vi "Write LINX I2C.vi"(8 "error in (no error)":errorcluster, 10 "LINX I2C":refnum<class "LINX I2C.lvclass">, 11 "BMP208 in":refnum<class "BMP208.lvclass">) -> (0 "error out":errorcluster, 3 "BMP208 out":refnum<class "BMP208.lvclass">)   [LabVIEW 2020, in "BMP208.lvclass"]
uses:
  BMP208.lvclass
  LINX I2C/LINX I2C.lvclass
  BMP208.lvclass/BMP208.ctl
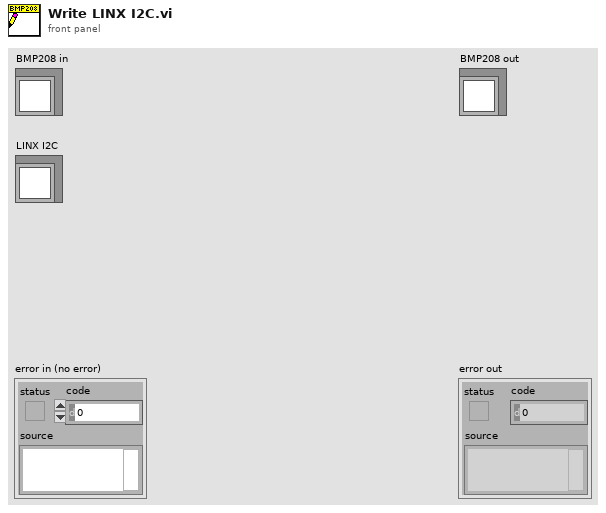
[diagram p1: front panel]
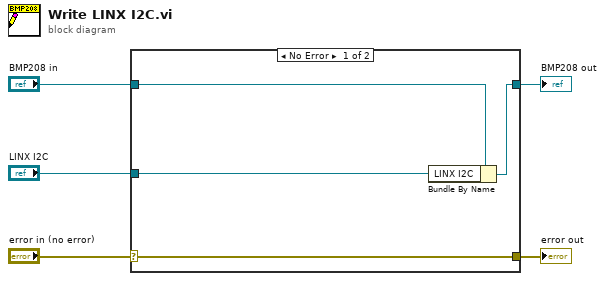
[diagram p0: block diagram]
diagram:
  n1 = case shown="No Error" "error in (no error)" {
    selector: "error in (no error)" -> [w9 w10]
    tunnel: [w9 w10] -> w4
    tunnel: [w7 w11] -> w2
    tunnel: "BMP208 in" -> [w8 w11]
    tunnel: "LINX I2C" -> [w6 _]
    frame No Error {
      n2 = Bundle By Name(cluster=w8, "LINX I2C"=w6) -> (w7:refnum<class "BMP208.lvclass">)
    }
    frame Error {
    }
  }
  "error out" <- w4
  "BMP208 out" <- w2
